vi "THERMOMETER using formula node.vi"() -> ()   [LabVIEW 2018]
panel:
  out "Thermometer":dbl(slide) scale=0.0..120.0
  out "?":bool
  in  "?":string
  in  "?":bool
  out "Max Temp (F)":dbl
  in  "S5":dbl
  in  "S4":dbl
  in  "S3":dbl
  in  "S2":dbl
  in  "S1":dbl
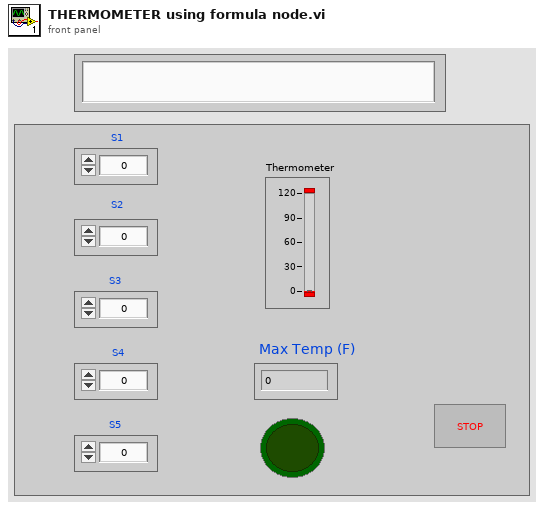
[diagram p1: front panel]
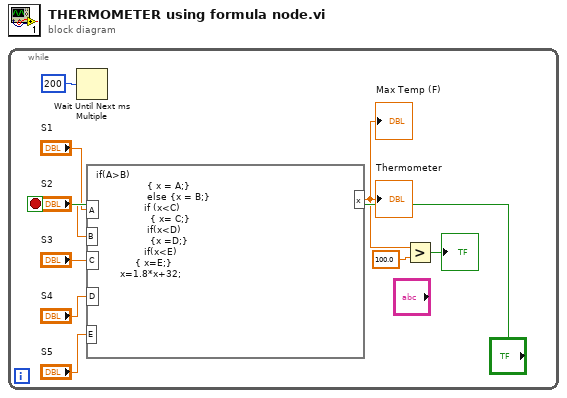
[diagram p0: block diagram]
diagram:
  n1 = while {
    stop <- "?" stop-if-true
    n2 = Wait Until Next ms Multiple(millisecond multiple=u32 200) -> ()  [unwired: 1 out]
    n3 = formula code="if(A>B)\n                 { x = A;}\n                 else {x = B;}\n                if (x<C)\n                  { x= C;}\n                 if(x<D)\n                  {x =D;}\n                if(x<E)\n             { x=E;}   \n        x=1.8*x+32;"("A"="S1", "B"="S2", "C"="S3", "D"="S4", "E"="S5") -> ("x"=w6:dbl)
    "Max Temp (F)" <- w6
    "Thermometer" <- w6
    n4 = Greater?(x=w6, y=100.0) -> (0:→"?":bool)
  }
